vi "ClassPanel.vi"(8 "error in (no error)":errorcluster caption="entrée d'erreur (pas d'erreur)", 11 "MultiHarp150.lvclass":refnum<class "MultiHarp150.lvclass">) -> (0 "error out":errorcluster caption="sortie d'erreur", 3 "MultiHarp150.lvclass Out":refnum<class "MultiHarp150.lvclass">)   [LabVIEW 2019, in "MultiHarp150.lvclass"]
uses:
  MultiHarp150.lvclass
  C:/Programmes Labview/LabscanV1A/DevicesClass/BaseDevice/BaseDevice.lvclass
  <userlib>/MultiHarp150/MH_InputChannel_LS.ctl
  <userlib>/MultiHarp150/MH_MeasMode.ctl
  <userlib>/MultiHarp150/MH_RefSource.ctl
  <userlib>/MultiHarp150/UIThread/MH_SetInpChanData.ctl
  <userlib>/MultiHarp150/UIThread/MH_SetInpChanCmds.ctl
  MultiHarp150.lvclass/MultiHarp150.ctl
  BaseDevice/ClassQueueMess.ctl
  MultiHarp150_Func.ctl
  BaseDevice/Accessor/GetClassEvent.vi
  <vilib>/Utility/error.llb/Error Cluster From Error Code.vi
  <vilib>/ErrorRing/Error Ring.xnode
panel:
  out "ClearRef":refnum<vi>
  in  "Con/Disc.":bool
  out "Rate Avg Data":i32[][](array[numeric])
  out "Avg ref":refnum<vi>
  out "RtGrphAct":bool
  out "ViRef":refnum<vi>
  out "Graph":refnum<vi>
  out "Dat":refnum<vi>
  out "Rate Data":i32[][](array[numeric])
  out "binsteps":i32
  out "SetInpChan":T1[](array[typedef])
  out "DevIdx":i32
  in  "MH Tabs":enum32{"Main", "Settings", "Channels"}(tab)
  in  "Halt":bool
  out "Timeleft (ms)":dbl=60.0 caption="TimeLeft(ms)"
  in  "Rd.Cnt\nAcqu.":bool
  in  "ClearGrp":bool
  in  "AcqOffset (ns)":i32 caption="Offset (ns)" min=-1000000 max=100000000 step=1
  in  "Acqu. Time (ms)":i32=60 min=1 step=1
  out "SyncRate (CPS)":i32=60 format="%^.0e"
  in  "Clear Graph":bool caption="Clear\nGraph"
  in  "Save Data":bool caption="Save\nHist."
  in  "AquireHist":bool caption="MiseAJour"
  in  "Contin.\nAcqu.":bool
  out "OverFlow":bool caption="Ovrflw:"
  out "Count Rates":i32[](array[numeric]) format="%#.0f"
  in  "Rate Graph":bool
  in  "Read Cont.":bool
  out "AllHistoStats":T3(array[cluster]) {"MaxTime 2" format="%.3e"; "MaxTime" format="%.3e"; "HistRate (CPS)" format="%#.3f"; "TotalCount" format="%#.1f"}
  in  "Stats Ch":u16(ring) caption="Ch" items=["1", "2", "3", "4", "Sum", ""]
  in  "Binning":T4(ring) caption="Resol. (ps)"
  in  "OvlLevel":u32=4294967295 caption="Overload.Lvl" min=1 step=1
  in  "Stop Ovl.":bool
  in  "HistoLength":T5(ring)=enum."65536" caption="Num Bins"
  in  "SyncDivider":i32(ring) caption="Divider" items=["1", "2", "4", "8", "16"]
  in  "SyncEdge":i32(ring) caption="Edge" items=["falling", "rising"]
  in  "SyncLevel":i32=-100 caption="Level (mV)" min=-1200 max=1200 step=1
  in  "SyncOffset":i32 caption="Offset (ps)" min=-100000 max=100000 step=5
  in  "UseDeadTime":bool caption="Use DT."
  in  "SyncDeadTime":i32=1000 caption="Dead T. (ps)" min=800 max=160000 step=1
  in  "Panel Refresh":u32=400 caption="Panel Refresh (ms)" min=200 max=10000 step=200
  in  "Ref Source":T6
  in  "Mode":T7 items=["HIST"=0, "T2"=2, "T3"=3]
  in  "Graph #":i32 min=0 max=256 step=1
  in  "Channels":T8[](array[typedef]) {"DeadTime" min=800 max=160000 step=1; "Edge" items=["falling", "rising"]; "Offset" min=-100000 max=100000 step=5; "Level" min=-1200 max=1200 step=1}
  in  "MainProgQ":refnum<queue>
  in  "MainProgQEvent":refnum<user-event>
  in  "Acq":bool
  in  "Stop":bool
  out "Init Program":bool
  # "MultiHarp 150"
  # "this MUST labeled with class name"
  # "this MUST be present and labeled \"Stop\" and \"Acq\""
  # "Single Acq"
  # "Sync Channel"
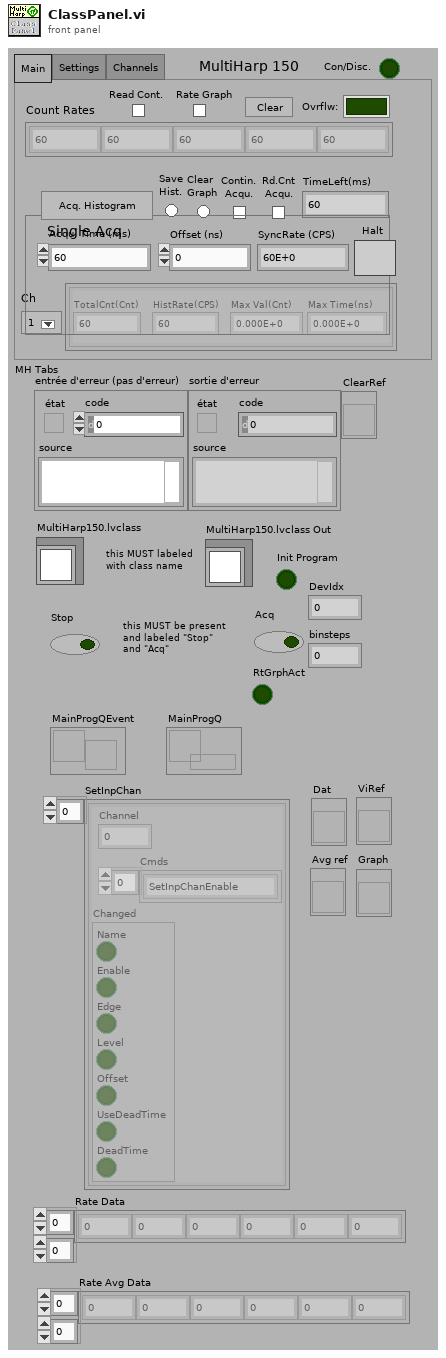
[diagram p1: front panel]
types:
  T1 = typedef "MH_SetInpChanData.ctl" = cluster{"Channel":i32, "Cmds":T2[], "Changed":cluster{"Name":bool, "Enable":bool, "Edge":bool, "Level":bool, "Offset":bool, "UseDeadTime":bool, "DeadTime":bool}}
  T2 = typedef "MH_SetInpChanCmds.ctl" = enum16{"SetInpChanEnable", "SetInpChanOffset", "SetInpChanDeadTime", "SetInpChanTrg"}
  T3 = cluster{"TotalCount":dbl, "HistRate (CPS)":dbl, "MaxTime 2":dbl, "MaxTime":dbl}[]
  T4 = enum16{"5", "10", "20", "40", "80", "160", "320", "640", "1280", "2560", "5120", "10240", "20480", "40960", "81920", "163840", "327680", "655360", "1310720", "2621440", "5242880", "10485760", "20971520", "41943040"}
  T5 = enum16{"1024", "2048", "4096", "8192", "16384", "32768", "65536"}
  T6 = typedef "MH_RefSource.ctl" = enum16{"INTERNAL", "EXTERNAL_10MHZ", "WR_MASTER_GENERIC", "WR_SLAVE_GENERIC", "WR_GRANDM_GENERIC", "EXTN_GPS_PPS", "EXTN_GPS_PPS_UART", "WR_MASTER_MHARP", "WR_SLAVE_MHARP", "WR_GRANDM_MHARP"}
  T7 = typedef "MH_MeasMode.ctl" = i32
  T8 = typedef "MH_InputChannel_LS.ctl" = cluster{"Name":string, "Enable":bool, "Edge":i32, "Level":i32, "Offset":i32, "UseDeadTime":bool, "DeadTime":i32}
  T9 = enum32{"Invalid", "Standard", "Closed", "Hidden", "Minimized", "Maximized"}
  T10 = typedef "MultiHarp150.lvclass/MultiHarp150_Func.ctl" = enum16{"ReadHistogram (Ph)", "ReadT2 (Ph)", "ReadT3 (Ph)", "ReadCount (Ph)"}
  T11 = enum16{"Enable", "Disable", "DisAndGrayed", "ReinitToDefVal", "EnumElementsArr"}
  T12 = cluster{dbl, "Panel Refresh":u32, "Rate Data Out":i32[][]}
  T13 = typedef "ClassQueueMess.ctl" = u16
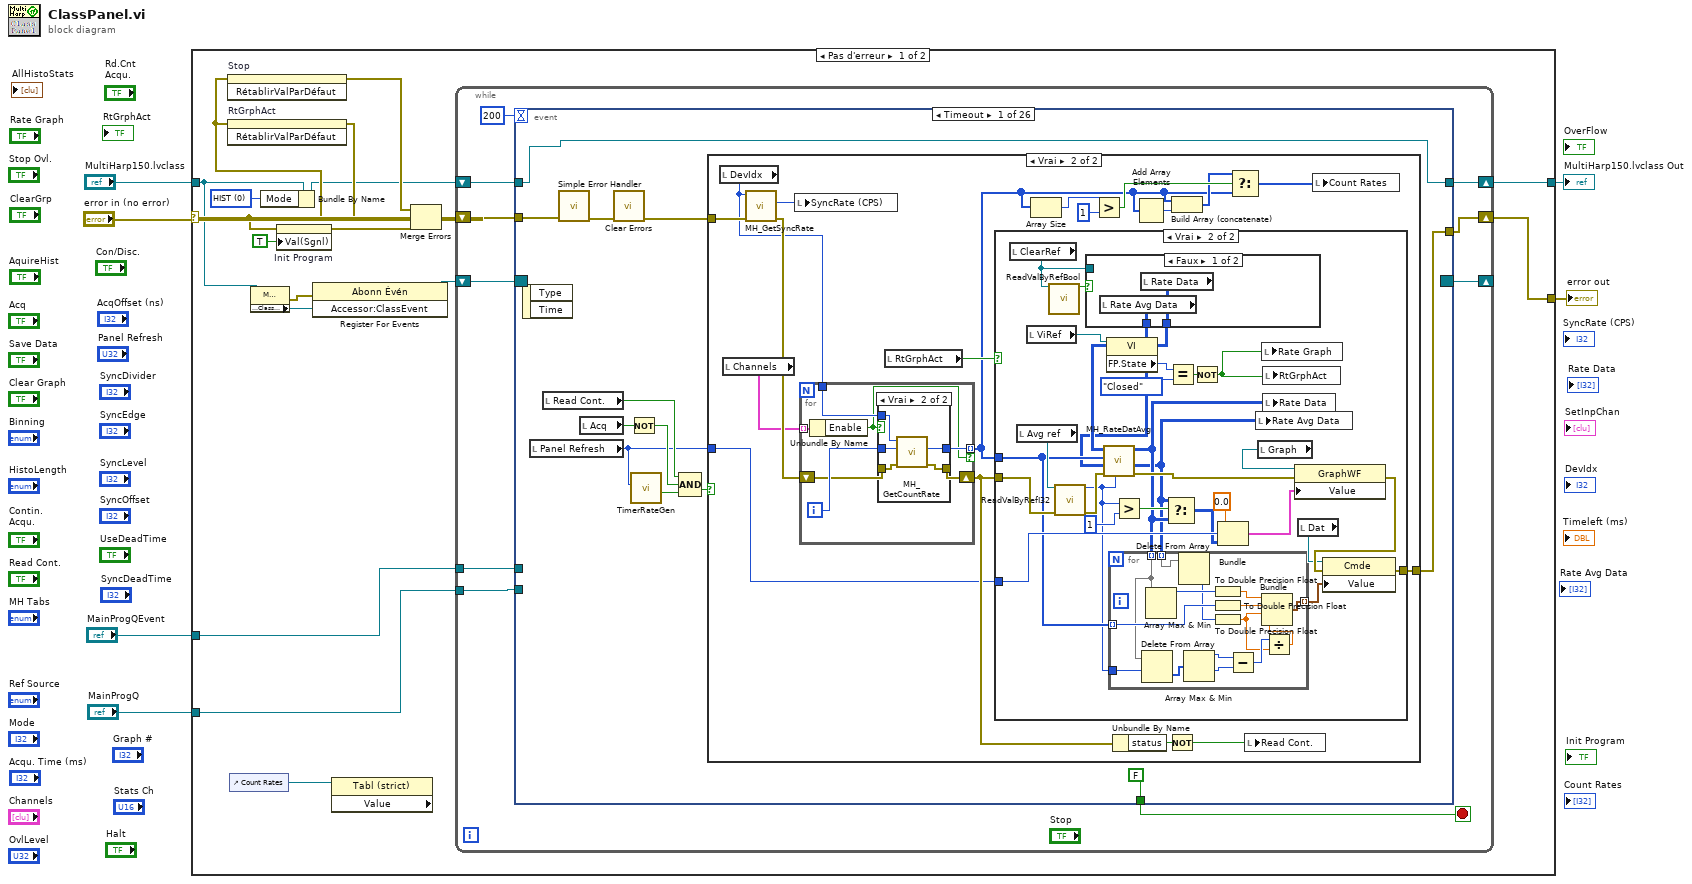
[diagram p0: block diagram]
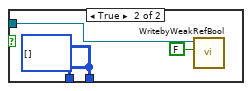
[diagram p4: hidden frame]
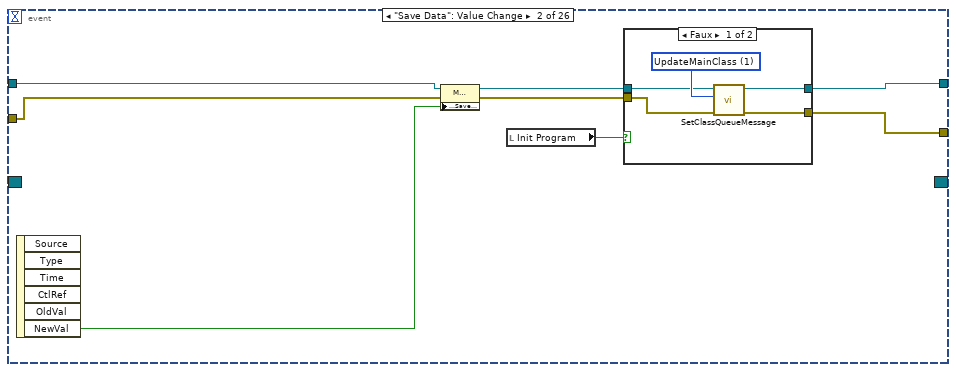
[diagram p6: hidden frame]
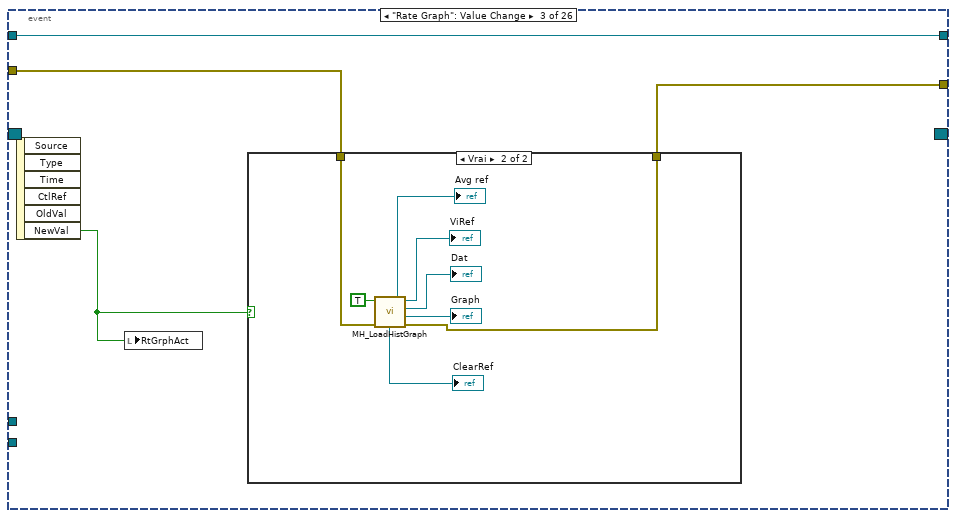
[diagram p8: hidden frame]
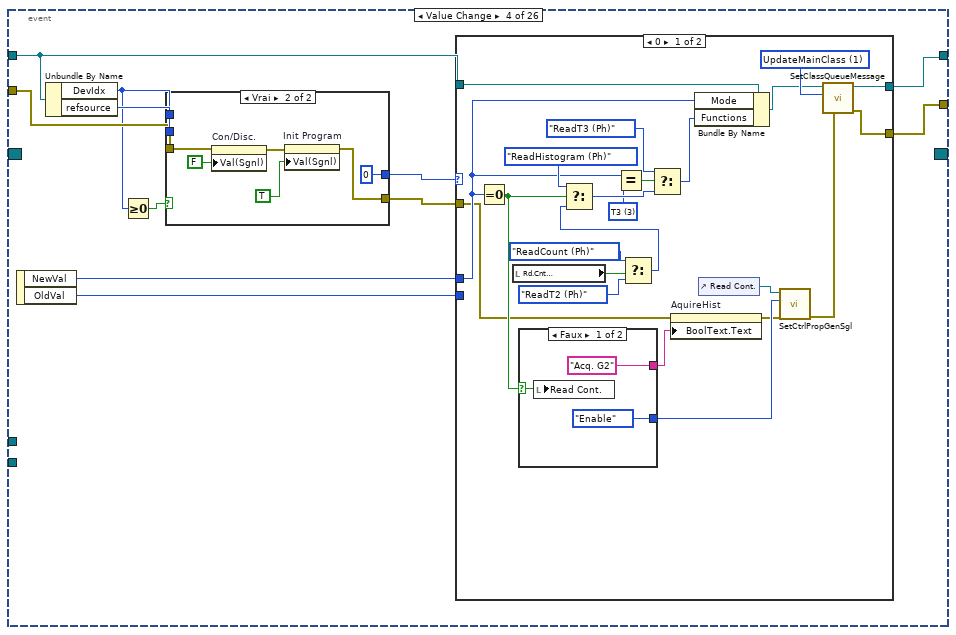
[diagram p10: hidden frame]
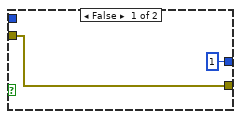
[diagram p11: hidden frame]
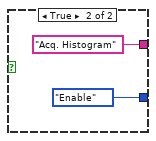
[diagram p12: hidden frame]
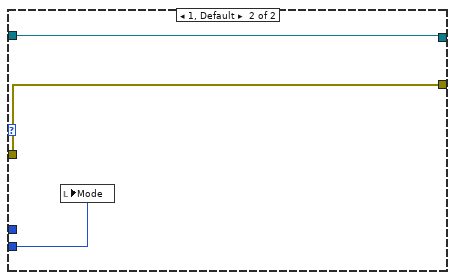
[diagram p13: hidden frame]
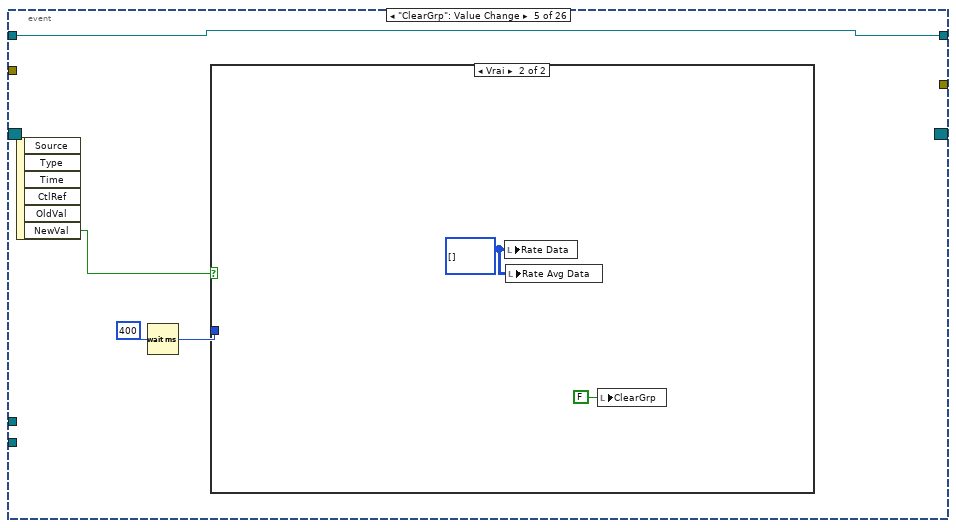
[diagram p14: hidden frame]
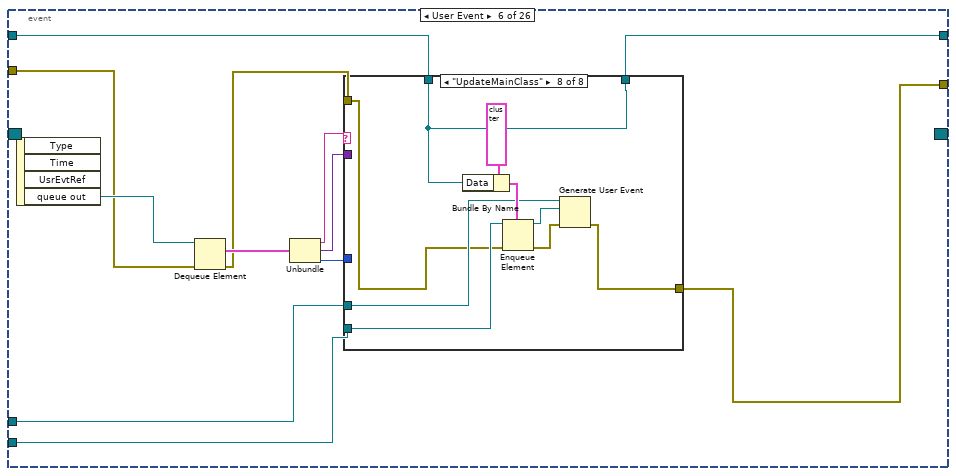
[diagram p16: hidden frame]
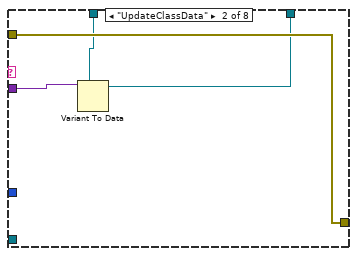
[diagram p18: hidden frame]
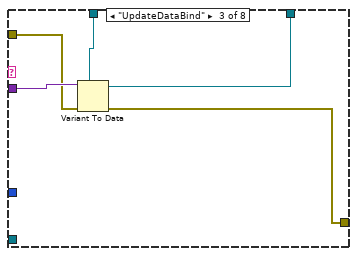
[diagram p19: hidden frame]
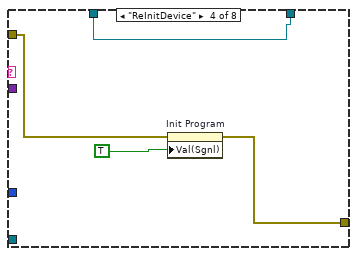
[diagram p20: hidden frame]
diagram:
  n1 = case shown="Pas d'erreur" "error in (no error)" {
    selector: "error in (no error)" -> [w11 w744]
    tunnel: [w23 w744] -> w5
    tunnel: "MultiHarp150.lvclass" -> [w19 w743]
    tunnel: [w22 w743] -> w3
    tunnel: "MainProgQEvent" -> [w17 _]
    tunnel: "MainProgQ" -> [w16 _]
    frame No Error {
      w8 = T7 0 items=["HIST"=0, "T2"=2, "T3"=3] ("Mode")
      n2 = invoke on="Stop" class="Bool (strict)" method="RétablirValParDéfaut"(error in=w11) -> (error out=w14:errorcluster)  [unwired: 2 in, 2 out]
      n3 = invoke on="RtGrphAct" class="Bool (strict)" method="RétablirValParDéfaut"(error in=w11) -> (error out=w13:errorcluster)  [unwired: 2 in, 2 out]
      n4 = control-ref of="Count Rates"() -> (w7:refnum<vi>)
      n5 = property class="MultiHarp150.lvclass"(reference=w19) -> (error out=w21:errorcluster, "Accessor:ClassEvent"=w20:refnum<user-event>)  [unwired: 1 in, 1 out]
      n6 = Bundle By Name(cluster=w19, "Mode"=w8) -> (w9:refnum<class "MultiHarp150.lvclass">)
      n7 = property on="Init Program" class="Bool (strict)"(error in=w11, "Val(Sgnl)"=TRUE ("Valeur (Signalisation)")) -> (error out=w10:errorcluster)  [unwired: 1 in, 1 out]
      n8 = register-events(error in=w21, w20) -> (reference out=w18:refnum<event-registration>)  [unwired: 1 in, 1 out]
      n9 = property class="Tabl (strict)" props=["Value"](reference=w7) -> ()  [unwired: 1 in, 3 out]
      n10 = Merge Errors(w14, w13, w10) -> (w15:errorcluster)
      n11 = while {
        shift-right: [w31] -> w23
        shift-left: w15 -> [w32]
        shift-right: [w29] -> w22
        shift-left: w9 -> [w30]
        shift-right: [w27] -> _
        shift-left: w18 -> [w28]
        tunnel: w17 -> [w26]
        tunnel: w16 -> [w25]
        stop <- w24 stop-if-true
        n12 = event shown="[0] Timeout" {
          selector: w28 -> [_ _ _ _ _ _ _ _ _ _ _ _ _ _ _ _ _ _ _ _ _ _ _ _ _ _]
          dyn-events: [_ _ _ _ _ _ _ _ _ _ _ _ _ _ _ _ _ _ _ _ _ _ _ _ _ _] -> w27
          timeout: 200 -> [_ _ _ _ _ _ _ _ _ _ _ _ _ _ _ _ _ _ _ _ _ _ _ _ _ _]
          tunnel: w32 -> [w44 w133 w144 w160 _ w212 w260 w316 w326 w346 w362 w380 w392 w410 _ w424 w488 w505 w535 w567 w591 w609 w625 w675 w702 w725]
          tunnel: [w41 w128 w143 w162 _ w216 w259 w315 w321 w341 w359 w373 w388 w413 _ w425 w489 w501 w531 w563 w586 w601 w624 w672 w704 w720] -> w31
          tunnel: w30 -> [w36 w134 w145 w155 w205 w222 w258 w317 w329 w347 w358 w381 w393 w408 w416 w427 w494 w496 w528 w560 w584 w600 w627 w674 w703 w726]
          tunnel: [FALSE _ _ _ _ _ _ _ _ _ _ _ _ _ _ _ _ _ _ _ _ _ _ TRUE FALSE _] -> w24
          tunnel: [w36 w129 w145 w164 w205 w215 w257 w314 w323 w343 w361 w375 w390 w414 w416 w421 w490 w502 w532 w565 w588 w606 w628 w673 w703 w719] -> w29
          tunnel: w26 -> [_ _ _ _ _ w214 _ _ _ _ _ _ _ _ _ _ _ _ _ _ _ _ w623 _ _ _]
          tunnel: w25 -> [_ _ _ _ _ w213 _ _ _ _ _ _ _ _ _ _ _ _ _ _ _ _ w622 _ _ _]
          event Timeout {
            n13 = event-data() -> ()  [unwired: 1 in, 2 out]
            n14 = local read "Panel Refresh"() -> (w35:u32)
            n15 = local read "Read Cont."() -> (w37:bool)
            n16 = call <vilib>:"Simple Error Handler.vi"("error in (no error)"=w44) -> ("error out"=w43:errorcluster)  [unwired: 4 in, 4 out]
            n17 = local read "Acq"() -> (w39:bool)
            n18 = call <vilib>:"Clear Errors.vi"("error in (no error)"=w43) -> ("error out"=w42:errorcluster)  [unwired: 5 in, 1 out]
            n19 = Not(x=w39) -> (.not. x?=w38:bool)
            n20 = call <userlib>:"TimerRateGen.vi"("Refresh(ms)"=w35) -> ("updated?"=w34:bool)  [unwired: 8 in, 2 out]
            n21 = Compound Arithmetic op=AND ("Opérateur arithmétique")(w37, w38, w34) -> (w40:bool)
            n22 = case shown="Vrai" w40 {
              tunnel: w42 -> [w46 w64]
              tunnel: [w46 w60] -> w41
              tunnel: w35 -> [_ w58]
              frame False {
              }
              frame True {
                n23 = local read "DevIdx"() -> (w48:i32)
                n24 = local read "Channels"() -> (w47:T8[])
                n25 = call <userlib>:"MH_GetSyncRate.vi"("error in (no error)"=w64, "devidx"=w48) -> ("error out"=w56:errorcluster, "syncrate"=w59:i32)  [unwired: 7 in, 1 out]
                n26 = local write "SyncRate (CPS)"(w59) -> ()
                n27 = for {
                  tunnel: w47 -> [w120] mode=indexing
                  tunnel: w48 -> [w118]
                  shift-right: [w116] -> w61
                  shift-left: w56 -> [w117]
                  tunnel: [w115] -> w50 mode=indexing if=w114
                  i -> [w119]
                  n28 = Unbundle By Name(w120) -> ("Enable"=w114:bool)
                  n29 = case shown="Vrai" w114 {
                    tunnel: w119 -> [_ w126]
                    tunnel: w118 -> [_ w122]
                    tunnel: w117 -> [w121 w125]
                    tunnel: [w121 w124] -> w116
                    tunnel: [_ w123] -> w115
                    frame False {
                    }
                    frame True {
                      n30 = call <userlib>:"MH_GetCountRate.vi"("error in (no error)"=w125, "Channel"=w126, "devidx"=w122) -> ("error out"=w124:errorcluster, "rate"=w123:i32)  [unwired: 6 in, 1 out]
                    }
                  }
                }
                n31 = local read "RtGrphAct"() -> (w57:bool)
                n32 = case shown="Vrai" w57 {
                  tunnel: w61 -> [w65 w79]
                  tunnel: [w65 w90] -> w60
                  tunnel: w50 -> [_ w77]
                  tunnel: w58 -> [_ w81]
                  frame False {
                  }
                  frame True {
                    n33 = local read "ClearRef"() -> (w71:refnum<vi>)
                    n34 = local read "Avg ref"() -> (w80:refnum<vi>)
                    n35 = local read "ViRef"() -> (w86:refnum<vi>)
                    n36 = call <userlib>:"ReadValByRefBool.vi"("Control Ref"=w71) -> ("Valeur"=w72:bool)  [unwired: 13 in, 1 out]
                    n37 = call <userlib>:"ReadValByRefI32.vi"("Control Ref"=w80, "error in"=w79) -> ("Valeur"=w66:i32, "error out"=w78:errorcluster)  [unwired: 12 in]
                    n38 = case shown="Faux" w72 {
                      tunnel: w71 -> [_ w96]
                      tunnel: [w95 w97] -> w69
                      tunnel: [w94 w97] -> w68
                      frame False {
                        n39 = local read "Rate Avg Data"() -> (w94:i32[][])
                        n40 = local read "Rate Data"() -> (w95:i32[][])
                      }
                      frame True {
                        w97 = i32[][] [] ("Rate Data")
                        n41 = call <userlib>:"WritebyWeakRefBool.vi"("Valeur"=FALSE, "Control Ref"=w96) -> ()  [unwired: 9 in, 1 out]
                      }
                    }
                    n42 = call <userlib>:"MH_RateDatAvg.vi"("Avg Val"=w66, "error in (no error)"=w78, "RateAvg Data"=w68, "Count Rates"=w77, "Rate Data"=w69) -> ("error out"=w76:errorcluster, "RateAvg Data Out"=w67:i32[][], "Rate Data Out"=w70:i32[][])  [unwired: 4 in]
                    n43 = property class="VI"(reference=w86) -> ("FP.State"=w85:T9)  [unwired: 1 in, 2 out]
                    n44 = for {
                      tunnel: w70 -> [w106] mode=indexing
                      tunnel: w77 -> [w110] mode=indexing
                      tunnel: [w113] -> w89 mode=indexing
                      tunnel: w67 -> [w108] mode=indexing
                      tunnel: w66 -> [w105]
                      n45 = Delete From Array(array=w106, length=w105) -> (deleted portion=w104:i32[])  [unwired: 1 in, 1 out]
                      n46 = Array Max & Min(array=w106) -> (max value=w109:i32)  [unwired: 3 out]
                      n47 = Delete From Array(array=w108) -> (deleted portion=w107:i32)  [unwired: 2 in, 1 out]
                      n48 = Array Max & Min(array=w104) -> (max value=w103:i32, min value=w102:i32)  [unwired: 2 out]
                      n49 = To Double Precision Float(number=w109) -> (double precision float=w112:dbl)
                      n50 = To Double Precision Float(number=w110) -> (double precision float=w111:dbl)
                      n51 = To Double Precision Float(number=w107) -> (double precision float=w100:dbl)
                      n52 = Subtract(x=w103, y=w102) -> (x-y=w101:i32)
                      n53 = Divide(x=w101, y=w100) -> (x/y=w99:dbl)
                      n54 = Bundle(w112, w111, w100, w99) -> (w113:cluster{dbl, dbl, dbl, dbl})  [unwired: 1 in]
                    }
                    n55 = Greater?(x=w66, y=1) -> (0:w74:bool)
                    n56 = Select(t=w67, s=w74, f=w70) -> (s? t:f=w73:i32[][])
                    n57 = Equal?(x=w85, y=T9."Closed") -> (x = y?=w83:bool)
                    n58 = Not(x=w83) -> (.not. x?=w82:bool)
                    n59 = Bundle(0.0, "Panel Refresh"=w81, "Rate Data Out"=w73) -> (w92:T12)  [unwired: 1 in]
                    n60 = local write "Rate Avg Data"(w67) -> ()
                    n61 = local read "Graph"() -> (w88:refnum<vi>)
                    n62 = local write "Rate Graph"(w82) -> ()
                    n63 = local write "RtGrphAct"(w82) -> ()
                    n64 = local write "Rate Data"(w70) -> ()
                    n65 = property class="GraphWF"(reference=w88, error in=w76, "Value"=w92) -> (error out=w91:errorcluster)  [unwired: 1 out]
                    n66 = local read "Dat"() -> (w87:refnum<vi>)
                    n67 = property class="Cmde"(reference=w87, error in=w91, "Value"=w89) -> (error out=w90:errorcluster)  [unwired: 1 out]
                  }
                }
                n68 = Array Size(array=w50) -> (size(s)=w55:i32)
                n69 = Greater?(x=w55, y=1) -> (0:w52:bool)
                n70 = Unbundle By Name(w61) -> ("status"=w63:bool)
                n71 = Add Array Elements(numeric array=w50) -> (sum=w53:i32)
                n72 = Not(x=w63) -> (.not. x?=w62:bool)
                n73 = Build Array (concatenate)(w50, w53) -> (w51:i32[])
                n74 = Select(t=w51, s=w52, f=w50) -> (s? t:f=w49:i32[])
                n75 = local write "Read Cont."(w62) -> ()
                n76 = local write "Count Rates"(w49) -> ()
              }
            }
          }
          event "Save Data": Value Change {
            n77 = event-data() -> ("NewVal"=w132:bool)  [unwired: 1 in, 5 out]
            n78 = property class="MultiHarp150.lvclass"(reference=w134, error in=w133, "Accessor:SaveArrDat"=w132) -> (reference out=w131:refnum<class "MultiHarp150.lvclass">, error out=w130:errorcluster)
            n79 = local read "Init Program"() -> (w127:bool)
            n80 = case shown="Faux" w127 {
              tunnel: w131 -> [w138 w141]
              tunnel: w130 -> [w137 w140]
              tunnel: [w136 w141] -> w129
              tunnel: [w135 w140] -> w128
              frame False {
                w139 = T13 1 items=["UpdateClassData", "UpdateMainClass"] ("Menu déroulant")
                n81 = call-dynamic "SetClassQueueMessage.vi"("ErrorIn(No Error)"=w137, "Menu déroulant"=w139, "DefaultDev.lvclass"=w138) -> ("sortie d'erreur"=w135:errorcluster, "DefaultDev.lvclass Out"=w136:refnum<class "MultiHarp150.lvclass">)  [unwired: 7 in]
              }
              frame True {
              }
            }
          }
          event "Rate Graph": Value Change {
            n82 = event-data() -> ("NewVal"=w142:bool)  [unwired: 1 in, 5 out]
            n83 = local write "RtGrphAct"(w142) -> ()
            n84 = case shown="Vrai" w142 {
              tunnel: w144 -> [w146 w152]
              tunnel: [w146 w151] -> w143
              frame False {
              }
              frame True {
                n85 = call <userlib>:"MH_LoadHistGraph.vi"("ErrIn(No Err)"=w152, "Rate Mode"=TRUE) -> ("ErrOut"=w151:errorcluster, "Graph"=→"Graph":refnum<vi>, "Dat"=→"Dat":refnum<vi>, "ViRef"=→"ViRef":refnum<vi>, "Avg ref"=→"Avg ref":refnum<vi>, "ClearRef"=→"ClearRef":refnum<vi>)  [unwired: 3 in, 1 out]
              }
            }
          }
          event Value Change {
            n86 = event-data() -> ("NewVal"=w158:T7, "OldVal"=w159:T7)  [unwired: 1 in]
            n87 = Unbundle By Name(w155) -> ("DevIdx"=w157:i32, "refsource"=w165:T6)
            n88 = Greater Or Equal To 0?(x=w157) -> (x >= 0?=w156:bool)
            n89 = case shown="Vrai" w156 {
              tunnel: w165 -> [_ _]
              tunnel: [w166 w169] -> w163
              tunnel: [1 ("return type") 0 ("return type")] -> w161
              tunnel: w157 -> [_ _]
              tunnel: w160 -> [w166 w173]
              frame False {
              }
              frame True {
                n90 = property on="Con/Disc." class="Bool (strict)"(error in=w173, "Val(Sgnl)"=FALSE ("Valeur (Signalisation)")) -> (error out=w171:errorcluster)  [unwired: 1 in, 1 out]
                n91 = property on="Init Program" class="Bool (strict)"(error in=w171, "Val(Sgnl)"=TRUE ("Valeur (Signalisation)")) -> (error out=w169:errorcluster)  [unwired: 1 in, 1 out]
              }
            }
            n92 = case shown="0" w161 {
              tunnel: w155 -> [w196 w204]
              tunnel: [w193 w204] -> w164
              tunnel: w163 -> [w179 w203]
              tunnel: [w192 w203] -> w162
              tunnel: w158 -> [w188 _]
              tunnel: w159 -> [_ w202]
              frame 0 {
                w187 = T7 3 items=["HIST"=0, "T2"=2, "T3"=3] ("y")
                w195 = T13 1 items=["UpdateClassData", "UpdateMainClass"] ("Menu déroulant")
                n93 = Equal To 0?(x=w188) -> (x = 0?=w183:bool)
                n94 = local read "Rd.Cnt\nAcqu."() -> (w177:bool)
                n95 = case shown="Faux" w183 {
                  selector: w183 -> [w199 _]
                  tunnel: [T11."Enable" ("Énum") T11."Enable" ("Énum")] -> w182
                  tunnel: ["Acq. G2" ("Texte booléen.Texte") "Acq. Histogram" ("Texte booléen.Texte")] -> w178
                  frame False {
                    n96 = local write "Read Cont."(w199) -> ()
                  }
                  frame True {
                  }
                }
                n97 = Equal?(x=w188, y=w187) -> (x = y?=w189:bool)
                n98 = Select(t=MultiHarp150_Func."ReadCount (Ph)" ("Functions"), s=w177, f=MultiHarp150_Func."ReadT2 (Ph)" ("Functions")) -> (s? t:f=w174:T10)
                n99 = Select(t=MultiHarp150_Func."ReadHistogram (Ph)" ("Functions"), s=w183, f=w174) -> (s? t:f=w190:T10)
                n100 = Select(t=MultiHarp150_Func."ReadT3 (Ph)" ("Functions"), s=w189, f=w190) -> (s? t:f=w185:T10)
                n101 = property on="AquireHist" class="Bool (strict)"(error in=w179, "BoolText.Text"=w178) -> (error out=w180:errorcluster)  [unwired: 1 in, 1 out]
                n102 = Bundle By Name(cluster=w196, "Mode"=w188, "Functions"=w185) -> (w194:refnum<class "MultiHarp150.lvclass">)
                n103 = control-ref of="Read Cont."() -> (w184:refnum<vi>)
                n104 = call <userlib>:"SetCtrlPropGenSgl.vi"("Error in"=w180, "Énum"=w182, "Controls"=w184) -> ("Error out"=w181:errorcluster)  [unwired: 3 in, 1 out]
                n105 = call-dynamic "SetClassQueueMessage.vi"("ErrorIn(No Error)"=w181, "Menu déroulant"=w195, "DefaultDev.lvclass"=w194) -> ("sortie d'erreur"=w192:errorcluster, "DefaultDev.lvclass Out"=w193:refnum<class "MultiHarp150.lvclass">)  [unwired: 7 in]
              }
              frame 1, Default {
                n106 = local write "Mode"(w202) -> ()
              }
            }
          }
          event "ClearGrp": Value Change {
            n107 = event-data() -> ("NewVal"=w208:bool)  [unwired: 1 in, 5 out]
            n108 = Wait (ms)(milliseconds to wait=u32 400 ("attente (ms)")) -> (millisecond timer value=w207:u32)
            n109 = case shown="Vrai" w208 {
              tunnel: w207 -> [_ _]
              frame False {
              }
              frame True {
                w209 = i32[][] [] ("Rate Data")
                n110 = local write "Rate Data"(w209) -> ()
                n111 = local write "Rate Avg Data"(w209) -> ()
                n112 = local write "ClearGrp"(FALSE ("ClearGrp")) -> ()
              }
            }
          }
          event User Event {
            n113 = event-data() -> ("queue out"=w220:refnum<queue>)  [unwired: 1 in, 3 out]
            n114 = Dequeue Element(queue=w220, error in (no error)=w212) -> (element=w221:cluster{"Message":string, "Data":variant, i32}, error out=w211:errorcluster)  [unwired: 1 in, 2 out]
            n115 = Unbundle(w221) -> ("Message"=w219:string, "Data"=w218:variant, w217:i32)
            n116 = case shown="\"UpdateMainClass\"" w219 {
              tunnel: w211 -> [w224 w228 w230 w235 w239 w242 w246 w249]
              tunnel: w218 -> [_ w227 w233 _ _ _ _ _]
              tunnel: w222 -> [w223 w226 w232 w237 w241 w243 w247 w252]
              tunnel: [w223 w225 w231 w237 w241 w243 w247 w252] -> w215
              tunnel: [w224 w228 w229 w234 w238 w242 w246 w248] -> w216
              tunnel: w217 -> [_ _ _ _ _ _ _ _]
              tunnel: w214 -> [_ _ _ _ _ _ _ w251]
              tunnel: w213 -> [_ _ _ _ _ _ _ w250]
              frame Default {
              }
              frame "UpdateClassData" {
                n117 = Variant To Data(type=w226, Variant=w227) -> (data=w225:refnum<class "MultiHarp150.lvclass">)  [unwired: 1 in, 1 out]
              }
              frame "UpdateDataBind" {
                n118 = Variant To Data(error in=w230, type=w232, Variant=w233) -> (data=w231:refnum<class "MultiHarp150.lvclass">, error out=w229:errorcluster)
              }
              frame "ReInitDevice" {
                n119 = property on="Init Program" class="Bool (strict)"(error in=w235, "Val(Sgnl)"=TRUE ("Valeur (Signalisation)")) -> (error out=w234:errorcluster)  [unwired: 1 in, 1 out]
              }
              frame "Disconnect Device" {
                n120 = property on="Con/Disc." class="Bool (strict)"(error in=w239, "Val(Sgnl)"=FALSE ("Valeur (Signalisation)")) -> (error out=w238:errorcluster)  [unwired: 1 in, 1 out]
              }
              frame "MeasDone" {
              }
              frame "ShowDiag" {
                n121 = control-ref of="This VI"() -> (w245:refnum<vi>)
                n122 = call <userlib>:"AnimExecGen.vi"("Animer l'exécution ?"=TRUE, "ViRef"=w245) -> ()  [unwired: 9 in, 1 out]
              }
              frame "UpdateMainClass" {
                n123 = Bundle By Name(cluster=cluster{"Message":string, "Data":variant, i32} {"Message"="", "Data"=variant, 0} ("élément"), "Data"=w252) -> (w253:cluster{"Message":string, "Data":variant, i32})
                n124 = Enqueue Element(queue=w250, element=w253, error in (no error)=w249) -> (queue out=w256:refnum<queue>, error out=w255:errorcluster)  [unwired: 1 in, 1 out]
                n125 = Generate User Event(user event=w251, event data cluster=w256, error in=w255) -> (error out=w248:errorcluster)  [unwired: 1 in, 1 out]
              }
            }
          }
          event "Init Program": Value Change {
            n126 = event-data() -> ("NewVal"=w261:bool)  [unwired: 1 in]
            n127 = case shown="Vrai" w261 {
              tunnel: w260 -> [w263 w302]
              tunnel: [w263 w289] -> w259
              tunnel: w258 -> [w262 w272]
              tunnel: [w262 w270] -> w257
              frame False {
              }
              frame True {
                n128 = xnode "Menu déroulant d'erreurs"() -> ("sortie d'erreur"=w266:errorcluster)
                n129 = Unbundle By Name(w272) -> ("Mode"=w286:T7, "refsource"=w284:T6, "Panel Refresh"=w285:dbl, "SyncDivider"=w281:i32, "SyncOffset"=w288:i32, "SyncEdge"=w296:i32, "SyncDeadTime"=w280:i32, "Binning"=w279:T4, "HistoLength"=w278:T5, "HistoOffset(ns)"=w275:i32, "OvlLevel"=w277:u32, "Channels"=w301:T8[], "SyncLevel"=w282:i32, "Stop Ovl."=w283:bool, "UseDeadTime"=w287:bool, "AcquTime(ms)"=w276:i32)
                n130 = for {
                  N: 8 -> [_]
                  tunnel: [w310] -> w265
                  tunnel: [w309] -> _
                  tunnel: [w311] -> w299
                  tunnel: w302 -> [w308]
                  i -> [w311]
                  stop <- w310 continue-if-true
                  n131 = call <userlib>:"MH_OpenDevice.vi"("error in (no error)"=w308, "devidx"=w311) -> ("error out"=w310:errorcluster, "serial"=w309:string)  [unwired: 7 in, 1 out]
                }
                n132 = local write "Mode"(w286) -> ()
                n133 = local write "Ref Source"(w284) -> ()
                n134 = local write "Panel Refresh"(w285) -> ()
                n135 = Select(t=w266, s=w265, f=w265) -> (s? t:f=w264:errorcluster)
                n136 = local write "SyncLevel"(w282) -> ()
                n137 = local write "Stop Ovl."(w283) -> ()
                n138 = local write "UseDeadTime"(w287) -> ()
                n139 = local write "Acqu. Time (ms)"(w276) -> ()
                n140 = local write "Channels"(w301) -> ()
                n141 = Select(t=-1, s=w264, f=w299) -> (s? t:f=w271:i32)
                n142 = call <userlib>:"MH_Initialize.vi"("error in (no error)"=w264, "refsource"=w284, "mode"=w286, "devidx"=w271) -> ("error out"=w269:errorcluster)  [unwired: 6 in, 1 out]
                n143 = property on="Save Data" class="Bool (strict)"(error in=w269, "Val(Sgnl)"=TRUE ("Valeur (Signalisation)")) -> (error out=w268:errorcluster)  [unwired: 1 in, 1 out]
                n144 = Bundle By Name(cluster=w272, "DevIdx"=w271) -> (w270:refnum<class "MultiHarp150.lvclass">)
                n145 = property on="SyncDivider" class="MDér (strict)"(error in=w268, "Val(Sgnl)"=w281) -> (error out=w295:errorcluster)  [unwired: 1 in, 1 out]
                n146 = property on="SyncOffset" class="NumNb (strict)"(error in=w295, "Val(Sgnl)"=w288) -> (error out=w294:errorcluster)  [unwired: 1 in, 1 out]
                n147 = property on="SyncEdge" class="MDér (strict)"(error in=w294, "Val(Sgnl)"=w296) -> (error out=w293:errorcluster)  [unwired: 1 in, 1 out]
                n148 = property on="SyncDeadTime" class="NumNb (strict)"(error in=w293, "Val(Sgnl)"=w280) -> (error out=w292:errorcluster)  [unwired: 1 in, 1 out]
                n149 = property on="SetInpChan" class="Tabl (strict)"(error in=w292, "Val(Sgnl)"=T1[] [{"Channel"=0, "Cmds"=[enum."SetInpChanEnable", enum."SetInpChanTrg", enum."SetInpChanOffset", enum."SetInpChanDeadTime"], "Changed"={"Name"=FALSE, "Enable"=FALSE, "Edge"=FALSE, "Level"=FALSE, "Offset"=FALSE, "UseDeadTime"=FALSE, "DeadTime"=FALSE}}, {"Channel"=1, "Cmds"=[enum."SetInpChanEnable", enum."SetInpChanTrg", enum."SetInpChanOffset", enum."SetInpChanDeadTime"], "Changed"={"Name"=FALSE, "Enable"=FALSE, "Edge"=FALSE, "Level"=FALSE, "Offset"=FALSE, "UseDeadTime"=FALSE, "DeadTime"=FALSE}}, {"Channel"=2, "Cmds"=[enum."SetInpChanEnable", enum."SetInpChanTrg", enum."SetInpChanOffset", enum."SetInpChanDeadTime"], "Changed"={"Name"=FALSE, "Enable"=FALSE, "Edge"=FALSE, "Level"=FALSE, "Offset"=FALSE, "UseDeadTime"=FALSE, "DeadTime"=FALSE}}, {"Channel"=3, "Cmds"=[enum."SetInpChanEnable", enum."SetInpChanTrg", enum."SetInpChanOffset", enum."SetInpChanDeadTime"], "Changed"={"Name"=FALSE, "Enable"=FALSE, "Edge"=FALSE, "Level"=FALSE, "Offset"=FALSE, "UseDeadTime"=FALSE, "DeadTime"=FALSE}}] ("Valeur (Signalisation)")) -> (error out=w291:errorcluster)  [unwired: 1 in, 1 out]
                n150 = property on="Binning" class="Énum (strict)"(error in=w291, "Val(Sgnl)"=w279) -> (error out=w290:errorcluster)  [unwired: 1 in, 1 out]
                n151 = property on="HistoLength" class="Énum (strict)"(error in=w290, "Val(Sgnl)"=w278) -> (error out=w274:errorcluster)  [unwired: 1 in, 1 out]
                n152 = property on="AcqOffset (ns)" class="NumNb (strict)"(error in=w274, "Val(Sgnl)"=w275) -> (error out=w273:errorcluster)  [unwired: 1 in, 1 out]
                n153 = property on="OvlLevel" class="NumNb (strict)"(error in=w273, "Val(Sgnl)"=w277) -> (error out=w289:errorcluster)  [unwired: 1 in, 1 out]
              }
            }
          }
          event "Panel Refresh": Value Change {
            w313 = T13 1 items=["UpdateClassData", "UpdateMainClass"] ("Menu déroulant")
            n154 = event-data() -> ("NewVal"=w318:u32)  [unwired: 1 in, 5 out]
            n155 = Bundle By Name(cluster=w317, "Panel Refresh"=w318) -> (w312:refnum<class "MultiHarp150.lvclass">)
            n156 = call-dynamic "SetClassQueueMessage.vi"("ErrorIn(No Error)"=w316, "Menu déroulant"=w313, "DefaultDev.lvclass"=w312) -> ("sortie d'erreur"=w315:errorcluster, "DefaultDev.lvclass Out"=w314:refnum<class "MultiHarp150.lvclass">)  [unwired: 7 in]
          }
          event "SyncDivider": Value Change {
            n157 = event-data() -> ("NewVal"=w320:i32)  [unwired: 1 in, 5 out]
            n158 = local read "DevIdx"() -> (w327:i32)
            n159 = Power Of 2(x=w320) -> (2^x=w330:dbl)
            n160 = To Long Integer(number=w330) -> (32bit integer=w328:i32)
            n161 = Bundle By Name(cluster=w329, "SyncDivider"=w320) -> (w324:refnum<class "MultiHarp150.lvclass">)
            n162 = call <userlib>:"MH_SetSyncDiv.vi"("error in (no error)"=w326, "SyncDivider"=w328, "devidx"=w327) -> ("error out"=w325:errorcluster)  [unwired: 7 in, 1 out]
            n163 = flat-sequence {
              tunnel: w325 -> [w338]
              tunnel: [w338] -> w322
              frame #0 {
                n164 = Wait (ms)(milliseconds to wait=u32 100) -> ()  [unwired: 1 out]
              }
            }
            n165 = local read "Init Program"() -> (w319:bool)
            n166 = case shown="Faux" w319 {
              tunnel: w324 -> [w334 w336]
              tunnel: [w333 w336] -> w323
              tunnel: w322 -> [w332 w337]
              tunnel: [w331 w337] -> w321
              frame False {
                w335 = T13 1 items=["UpdateClassData", "UpdateMainClass"] ("Menu déroulant")
                n167 = call-dynamic "SetClassQueueMessage.vi"("ErrorIn(No Error)"=w332, "Menu déroulant"=w335, "DefaultDev.lvclass"=w334) -> ("sortie d'erreur"=w331:errorcluster, "DefaultDev.lvclass Out"=w333:refnum<class "MultiHarp150.lvclass">)  [unwired: 7 in]
              }
              frame True {
              }
            }
          }
          event "SyncOffset": Value Change {
            n168 = event-data() -> ("NewVal"=w345:i32)  [unwired: 1 in]
            n169 = local read "DevIdx"() -> (w348:i32)
            n170 = call <userlib>:"MH_SetSyncChannelOffset.vi"("error in (no error)"=w346, "Offset"=w345, "devidx"=w348) -> ("error out"=w342:errorcluster)  [unwired: 7 in, 1 out]
            n171 = Bundle By Name(cluster=w347, "SyncOffset"=w345) -> (w344:refnum<class "MultiHarp150.lvclass">)
            n172 = local read "Init Program"() -> (w340:bool)
            n173 = case shown="Faux" w340 {
              tunnel: w344 -> [w352 w354]
              tunnel: [w351 w354] -> w343
              tunnel: w342 -> [w350 w355]
              tunnel: [w349 w355] -> w341
              frame False {
                w353 = T13 1 items=["UpdateClassData", "UpdateMainClass"] ("Menu déroulant")
                n174 = call-dynamic "SetClassQueueMessage.vi"("ErrorIn(No Error)"=w350, "Menu déroulant"=w353, "DefaultDev.lvclass"=w352) -> ("sortie d'erreur"=w349:errorcluster, "DefaultDev.lvclass Out"=w351:refnum<class "MultiHarp150.lvclass">)  [unwired: 7 in]
              }
              frame True {
              }
            }
          }
          event "SyncEdge": Value Change {
            n175 = event-data() -> ("NewVal"=w363:i32)  [unwired: 1 in]
            n176 = local read "SyncLevel"() -> (w364:i32)
            n177 = local read "DevIdx"() -> (w365:i32)
            n178 = call <userlib>:"MH_SetSyncEdgeTrg.vi"("error in (no error)"=w362, "edge"=w363, "level"=w364, "devidx"=w365) -> ("error out"=w360:errorcluster)  [unwired: 6 in, 1 out]
            n179 = Bundle By Name(cluster=w358, "SyncEdge"=w363) -> (w357:refnum<class "MultiHarp150.lvclass">)
            n180 = local read "Init Program"() -> (w356:bool)
            n181 = case shown="Faux" w356 {
              tunnel: [w369 w372] -> w361
              tunnel: w360 -> [w368 w371]
              tunnel: [w367 w371] -> w359
              tunnel: w357 -> [w366 w372]
              frame False {
                w370 = T13 1 items=["UpdateClassData", "UpdateMainClass"] ("Menu déroulant")
                n182 = call-dynamic "SetClassQueueMessage.vi"("ErrorIn(No Error)"=w368, "Menu déroulant"=w370, "DefaultDev.lvclass"=w366) -> ("sortie d'erreur"=w367:errorcluster, "DefaultDev.lvclass Out"=w369:refnum<class "MultiHarp150.lvclass">)  [unwired: 7 in]
              }
              frame True {
              }
            }
          }
          event "SyncLevel": Value Change {
            w377 = T13 1 items=["UpdateClassData", "UpdateMainClass"] ("Menu déroulant")
            n183 = event-data() -> ("NewVal"=w378:i32)  [unwired: 1 in]
            n184 = local read "SyncEdge"() -> (w379:i32)
            n185 = local read "DevIdx"() -> (w382:i32)
            n186 = call <userlib>:"MH_SetSyncEdgeTrg.vi"("error in (no error)"=w380, "edge"=w379, "level"=w378, "devidx"=w382) -> ("error out"=w374:errorcluster)  [unwired: 6 in, 1 out]
            n187 = Bundle By Name(cluster=w381, "SyncLevel"=w378) -> (w376:refnum<class "MultiHarp150.lvclass">)
            n188 = call-dynamic "SetClassQueueMessage.vi"("ErrorIn(No Error)"=w374, "Menu déroulant"=w377, "DefaultDev.lvclass"=w376) -> ("sortie d'erreur"=w373:errorcluster, "DefaultDev.lvclass Out"=w375:refnum<class "MultiHarp150.lvclass">)  [unwired: 7 in]
          }
          event "SyncDeadTime": Value Change {
            n189 = event-data() -> ("NewVal"=w386:i32)  [unwired: 1 in]
            n190 = local read "UseDeadTime"() -> (w385:bool)
            n191 = local read "DevIdx"() -> (w394:i32)
            n192 = Boolean To (0,1)(Boolean=w385) -> (0, 1=w387:i16)
            n193 = To Long Integer(number=w387) -> (32bit integer=w384:i32)
            n194 = call <userlib>:"MH_SetSyncDeadTime.vi"("error in (no error)"=w392, "deadtime"=w386, "on"=w384, "devidx"=w394) -> ("error out"=w389:errorcluster)  [unwired: 6 in, 1 out]
            n195 = Bundle By Name(cluster=w393, "SyncDeadTime"=w386) -> (w391:refnum<class "MultiHarp150.lvclass">)
            n196 = local read "Init Program"() -> (w383:bool)
            n197 = case shown="Faux" w383 {
              tunnel: w391 -> [w398 w400]
              tunnel: [w397 w400] -> w390
              tunnel: w389 -> [w396 w401]
              tunnel: [w395 w401] -> w388
              frame False {
                w399 = T13 1 items=["UpdateClassData", "UpdateMainClass"] ("Menu déroulant")
                n198 = call-dynamic "SetClassQueueMessage.vi"("ErrorIn(No Error)"=w396, "Menu déroulant"=w399, "DefaultDev.lvclass"=w398) -> ("sortie d'erreur"=w395:errorcluster, "DefaultDev.lvclass Out"=w397:refnum<class "MultiHarp150.lvclass">)  [unwired: 7 in]
              }
              frame True {
              }
            }
          }
          event "Channels": Value Change {
            w415 = T13 1 items=["UpdateClassData", "UpdateMainClass"] ("Menu déroulant")
            n199 = event-data() -> ("OldVal"=w412:T8[], "NewVal"=w411:T8[])  [unwired: 1 in, 4 out]
            n200 = call <userlib>:"MH_SetInputChannels.vi"("error in (no error)"=w410, "Channels new"=w411, "Channels old"=w412) -> ("error out"=w409:errorcluster, "SetInpChan"=w405:T1[], "Channels"=w406:T8[])  [unwired: 6 in]
            n201 = Bundle By Name(cluster=w408, "Channels"=w406) -> (w407:refnum<class "MultiHarp150.lvclass">)
            n202 = local write "Channels"(w406) -> ()
            n203 = property on="SetInpChan" class="Tabl (strict)"(error in=w409, "Val(Sgnl)"=w405) -> (error out=w404:errorcluster)  [unwired: 1 in, 1 out]
            n204 = call "SetHistDataName.vi"("error in (no error)"=w404, "SetInpChan"=w405, "Channels"=w406, "MultiHarp150.lvclass"=w407) -> ("error out"=w403:errorcluster, "MultiHarp150.lvclass Out"=w402:refnum<class "MultiHarp150.lvclass">)  [unwired: 6 in]
            n205 = call-dynamic "SetClassQueueMessage.vi"("ErrorIn(No Error)"=w403, "Menu déroulant"=w415, "DefaultDev.lvclass"=w402) -> ("sortie d'erreur"=w413:errorcluster, "DefaultDev.lvclass Out"=w414:refnum<class "MultiHarp150.lvclass">)  [unwired: 7 in]
          }
          event "Stats Ch": Value Change {
            n206 = event-data() -> ("NewVal"=w418:u16)  [unwired: 1 in, 5 out]
            n207 = Build Array(w418) -> (w417:u16[])
            n208 = property on="AllHistoStats" class="Tabl (strict)"("Index Values"=w417) -> ()  [unwired: 2 in, 2 out]
          }
          event "SetInpChan": Value Change {
            n209 = event-data() -> ("NewVal"=w426:T1[])  [unwired: 1 in]
            n210 = local read "Channels"() -> (w429:T8[])
            n211 = local read "DevIdx"() -> (w431:i32)
            n212 = Empty Array?(array=w429) -> (empty?=w428:bool)
            n213 = Select(t=T8[] [{"Name"="Ch.1", "Enable"=FALSE, "Edge"=0, "Level"=-150, "Offset"=0, "UseDeadTime"=FALSE, "DeadTime"=800}, {"Name"="Ch.2", "Enable"=FALSE, "Edge"=0, "Level"=-150, "Offset"=0, "UseDeadTime"=FALSE, "DeadTime"=800}, {"Name"="Ch.3", "Enable"=FALSE, "Edge"=0, "Level"=-150, "Offset"=0, "UseDeadTime"=FALSE, "DeadTime"=800}, {"Name"="Ch.4", "Enable"=FALSE, "Edge"=0, "Level"=-150, "Offset"=0, "UseDeadTime"=FALSE, "DeadTime"=800}] ("Channels"), s=w428, f=w429) -> (s? t:f=w422:T8[])
            n214 = case shown="Vrai" w428 {
              tunnel: w427 -> [w441 w444]
              tunnel: [w441 w443] -> w423
              tunnel: w422 -> [_ w442]
              frame False {
              }
              frame True {
                n215 = Bundle By Name(cluster=w444, "Channels"=w442) -> (w443:refnum<class "MultiHarp150.lvclass">)
                n216 = local write "Channels"(w442) -> ()
              }
            }
            n217 = for {
              tunnel: w426 -> [w448] mode=indexing
              shift-right: [w452] -> w432
              shift-left: w424 -> [w451]
              tunnel: w422 -> [w450]
              tunnel: w431 -> [w449]
              n218 = Unbundle By Name(w448) -> ("Cmds"=w447:T2[], "Channel"=w445:i32)
              n219 = Index Array(array=w450, index=w445) -> (element=w446:T8)
              n220 = for {
                tunnel: w445 -> [w458]
                tunnel: w446 -> [w455]
                tunnel: w449 -> [w454]
                tunnel: w447 -> [w453] mode=indexing
                shift-right: [w457] -> w452
                shift-left: w451 -> [w456]
                n221 = case shown="\"SetInpChanDeadTime\"" w453 {
                  tunnel: w458 -> [_ w463 w467 w473 w483]
                  tunnel: [w459 w460 w470 w475 w481] -> w457
                  tunnel: w456 -> [w459 w461 w469 w472 w482]
                  tunnel: w455 -> [_ w465 w471 w480 w487]
                  tunnel: w454 -> [_ w464 w466 w474 w486]
                  frame Default {
                  }
                  frame "SetInpChanEnable" {
                    n222 = Unbundle By Name(w465) -> ("Enable"=w462:bool)
                    n223 = call <userlib>:"MH_SetInputChannelEnable.vi"("error in (no error)"=w461, "enable"=w462, "channel"=w463, "devidx"=w464) -> ("error out"=w460:errorcluster)  [unwired: 6 in, 1 out]
                  }
                  frame "SetInpChanOffset" {
                    n224 = Unbundle By Name(w471) -> ("Offset"=w468:i32)
                    n225 = call <userlib>:"MH_SetInputChannelOffset.vi"("error in (no error)"=w469, "Offset"=w468, "channel"=w467, "devidx"=w466) -> ("error out"=w470:errorcluster)  [unwired: 6 in, 1 out]
                  }
                  frame "SetInpChanDeadTime" {
                    n226 = Unbundle By Name(w480) -> ("UseDeadTime"=w479:bool, "DeadTime"=w476:i32)
                    n227 = Boolean To (0,1)(Boolean=w479) -> (0, 1=w478:i16)
                    n228 = To Long Integer(number=w478) -> (32bit integer=w477:i32)
                    n229 = call <userlib>:"MH_SetInputDeadTime.vi"("channel"=w473, "error in (no error)"=w472, "deadtime"=w476, "on"=w477, "devidx"=w474) -> ("error out"=w475:errorcluster)  [unwired: 5 in, 1 out]
                  }
                  frame "SetInpChanTrg" {
                    n230 = Unbundle By Name(w487) -> ("Level"=w485:i32, "Edge"=w484:i32)
                    n231 = call <userlib>:"MH_SetInputEdgeTrg.vi"("channel"=w483, "error in (no error)"=w482, "edge"=w484, "level"=w485, "devidx"=w486) -> ("error out"=w481:errorcluster)  [unwired: 5 in, 1 out]
                  }
                }
              }
            }
            n232 = local read "Init Program"() -> (w419:bool)
            n233 = case shown="Vrai" w419 {
              tunnel: w424 -> [w433 w440]
              tunnel: w423 -> [w434 w439]
              tunnel: w422 -> [_ w438]
              tunnel: [w434 w437] -> w421
              tunnel: [w433 w436] -> w420
              frame False {
              }
              frame True {
                n234 = call "SetHistDataName.vi"("ForceSet"=TRUE, "error in (no error)"=w440, "Channels"=w438, "MultiHarp150.lvclass"=w439) -> ("error out"=w436:errorcluster, "MultiHarp150.lvclass Out"=w437:refnum<class "MultiHarp150.lvclass">)  [unwired: 6 in]
              }
            }
            n235 = Merge Errors(w420, w432) -> (w425:errorcluster)
          }
          event "Acqu. Time (ms)": Value Change {
            w492 = T13 1 items=["UpdateClassData", "UpdateMainClass"] ("Menu déroulant")
            n236 = event-data() -> ("NewVal"=w493:i32)  [unwired: 1 in, 5 out]
            n237 = Bundle By Name(cluster=w494, "AcquTime(ms)"=w493) -> (w491:refnum<class "MultiHarp150.lvclass">)
            n238 = call-dynamic "SetClassQueueMessage.vi"("ErrorIn(No Error)"=w488, "Menu déroulant"=w492, "DefaultDev.lvclass"=w491) -> ("sortie d'erreur"=w489:errorcluster, "DefaultDev.lvclass Out"=w490:refnum<class "MultiHarp150.lvclass">)  [unwired: 7 in]
          }
          event "Binning": Value Change {
            n239 = event-data() -> ("NewVal"=w504:T4)  [unwired: 1 in]
            n240 = To Long Integer(number=w504) -> (32bit integer=w500:i32)
            n241 = local read "DevIdx"() -> (w498:i32)
            n242 = Unbundle By Name(w496) -> ("Mode"=w495:T7)
            n243 = case shown="1, Par défaut" w495 {
              tunnel: w496 -> [w506 w519]
              tunnel: w505 -> [w507 w518]
              tunnel: [w506 w517] -> w503
              tunnel: w500 -> [_ w515]
              tunnel: [w507 w513] -> w499
              tunnel: w498 -> [_ w512]
              frame 1, Default {
                # "Prop Not ValiD in g(t) MODE"
              }
              frame 0 {
                n244 = call <userlib>:"MH_SetBinning.vi"("error in (no error)"=w518, "Binning"=w515, "devidx"=w512) -> ("error out"=w516:errorcluster, "return type"=w514:i32)  [unwired: 7 in]
                n245 = call <userlib>:"MH_GetBaseResolution.vi"("error in (no error)"=w516, "devidx"=w512) -> ("error out"=w513:errorcluster, "binsteps"=→"binsteps":i32, "resolution"=w510:dbl)  [unwired: 6 in, 1 out]
                n246 = Divide(x=w510, y=1000.0) -> (x/y=w509:dbl)
                n247 = Bundle By Name(cluster=w519, "Binning"=w514, "Resolution (ns)"=w509) -> (w517:refnum<class "MultiHarp150.lvclass">)
              }
            }
            n248 = local read "Init Program"() -> (w497:bool)
            n249 = case shown="Faux" w497 {
              tunnel: w503 -> [w523 w526]
              tunnel: [w522 w526] -> w502
              tunnel: [w521 w525] -> w501
              tunnel: w499 -> [w520 w525]
              frame False {
                w524 = T13 1 items=["UpdateClassData", "UpdateMainClass"] ("Menu déroulant")
                n250 = call-dynamic "SetClassQueueMessage.vi"("ErrorIn(No Error)"=w520, "Menu déroulant"=w524, "DefaultDev.lvclass"=w523) -> ("sortie d'erreur"=w521:errorcluster, "DefaultDev.lvclass Out"=w522:refnum<class "MultiHarp150.lvclass">)  [unwired: 7 in]
              }
              frame True {
              }
            }
          }
          event "HistoLength": Value Change {
            n251 = event-data() -> ("NewVal"=w534:T5)  [unwired: 1 in]
            n252 = local read "DevIdx"() -> (w536:i32)
            n253 = Unbundle By Name(w528) -> ("Mode"=w527:T7)
            n254 = case shown="0" w527 {
              tunnel: w536 -> [_ w549]
              tunnel: w528 -> [w538 w548]
              tunnel: w535 -> [w537 w547]
              tunnel: w534 -> [_ w546]
              tunnel: [w538 w545] -> w533
              tunnel: [w537 w539] -> w529
              frame 1, Default {
                # "Prop Not ValiD in g(t) MODE"
              }
              frame 0 {
                n255 = To Long Integer(number=w546) -> (32bit integer=w544:i32)
                n256 = call <userlib>:"MH_SetHistoLen.vi"("error in (no error)"=w547, "lencode"=w544, "devidx"=w549) -> ("error out"=w540:errorcluster, "actuallen"=w542:i32)  [unwired: 6 in, 1 out]
                n257 = for {
                  N: w542 -> [_]
                  tunnel: [w550] -> w541 mode=indexing
                  i -> [w551]
                  n258 = To Double Precision Float(number=w551) -> (double precision float=w550:dbl)
                }
                n259 = property class="MultiHarp150.lvclass"(reference=w548, error in=w540, "Accessor:ScanTable"=w541) -> (reference out=w543:refnum<class "MultiHarp150.lvclass">, error out=w539:errorcluster)
                n260 = Bundle By Name(cluster=w543, "HistoLength"=w546, "Actual_H_Lenght(bin)"=w542) -> (w545:refnum<class "MultiHarp150.lvclass">)
              }
            }
            n261 = local read "Init Program"() -> (w530:bool)
            n262 = case shown="Faux" w530 {
              tunnel: w533 -> [w555 w558]
              tunnel: [w554 w558] -> w532
              tunnel: w529 -> [w553 w557]
              tunnel: [w552 w557] -> w531
              frame False {
                w556 = T13 1 items=["UpdateClassData", "UpdateMainClass"] ("Menu déroulant")
                n263 = call-dynamic "SetClassQueueMessage.vi"("ErrorIn(No Error)"=w553, "Menu déroulant"=w556, "DefaultDev.lvclass"=w555) -> ("sortie d'erreur"=w552:errorcluster, "DefaultDev.lvclass Out"=w554:refnum<class "MultiHarp150.lvclass">)  [unwired: 7 in]
              }
              frame True {
              }
            }
          }
          event "AcqOffset (ns)": Value Change {
            n264 = event-data() -> ("NewVal"=w561:i32)  [unwired: 1 in]
            n265 = Unbundle By Name(w560) -> ("Mode"=w559:T7)
            n266 = case shown="1, Par défaut" w559 {
              tunnel: w560 -> [w569 w574]
              tunnel: w567 -> [w568 w573]
              tunnel: [w569 w572] -> w566
              tunnel: [w568 w571] -> w564
              tunnel: w561 -> [_ w570]
              frame 1, Default {
                # "Prop Not ValiD in g(t) MODE"
              }
              frame 0 {
                n267 = local read "DevIdx"() -> (w575:i32)
                n268 = Bundle By Name(cluster=w574, "HistoOffset(ns)"=w570) -> (w572:refnum<class "MultiHarp150.lvclass">)
                n269 = call <userlib>:"MH_SetOffset.vi"("error in (no error)"=w573, "Offset"=w570, "devidx"=w575) -> ("error out"=w571:errorcluster)  [unwired: 7 in, 1 out]
              }
            }
            n270 = local read "Init Program"() -> (w562:bool)
            n271 = case shown="Faux" w562 {
              tunnel: w566 -> [w579 w582]
              tunnel: [w578 w582] -> w565
              tunnel: w564 -> [w577 w581]
              tunnel: [w576 w581] -> w563
              frame False {
                w580 = T13 1 items=["UpdateClassData", "UpdateMainClass"] ("Menu déroulant")
                n272 = call-dynamic "SetClassQueueMessage.vi"("ErrorIn(No Error)"=w577, "Menu déroulant"=w580, "DefaultDev.lvclass"=w579) -> ("sortie d'erreur"=w576:errorcluster, "DefaultDev.lvclass Out"=w578:refnum<class "MultiHarp150.lvclass">)  [unwired: 7 in]
              }
              frame True {
              }
            }
          }
          event "Stop Ovl.": Value Change {
            w590 = T13 1 items=["UpdateClassData", "UpdateMainClass"] ("Menu déroulant")
            n273 = event-data() -> ("NewVal"=w585:bool)  [unwired: 1 in]
            n274 = local read "DevIdx"() -> (w592:i32)
            n275 = Unbundle By Name(w584) -> ("Mode"=w583:T7)
            n276 = case shown="1, Par défaut" w583 {
              tunnel: w592 -> [w597 _]
              tunnel: w591 -> [w596 w598]
              tunnel: [w595 w598] -> w587
              tunnel: w585 -> [w594 _]
              frame 0 {
                n277 = local read "OvlLevel"() -> (w593:u32)
                n278 = call <userlib>:"MH_SetStopOverflow.vi"("error in (no error)"=w596, "stopcount"=w593, "StopOnOverflow"=w594, "devidx"=w597) -> ("error out"=w595:errorcluster)  [unwired: 6 in, 1 out]
              }
              frame 1, Default {
                # "Prop Not ValiD in g(t) MODE"
              }
            }
            n279 = Bundle By Name(cluster=w584, "Stop Ovl."=w585) -> (w589:refnum<class "MultiHarp150.lvclass">)
            n280 = call-dynamic "SetClassQueueMessage.vi"("ErrorIn(No Error)"=w587, "Menu déroulant"=w590, "DefaultDev.lvclass"=w589) -> ("sortie d'erreur"=w586:errorcluster, "DefaultDev.lvclass Out"=w588:refnum<class "MultiHarp150.lvclass">)  [unwired: 7 in]
          }
          event "OvlLevel": Value Change {
            w608 = T13 1 items=["UpdateClassData", "UpdateMainClass"] ("Menu déroulant")
            n281 = event-data() -> ("NewVal"=w604:u32)  [unwired: 1 in]
            n282 = Unbundle By Name(w600) -> ("Mode"=w599:T7)
            n283 = case shown="0" w599 {
              tunnel: w609 -> [w610 w614]
              tunnel: [w610 w613] -> w605
              tunnel: w604 -> [_ w612]
              frame 1, Default {
              }
              frame 0 {
                n284 = local read "UseDeadTime"() -> (w611:bool)
                n285 = local read "DevIdx"() -> (w615:i32)
                n286 = call <userlib>:"MH_SetStopOverflow.vi"("error in (no error)"=w614, "stopcount"=w612, "StopOnOverflow"=w611, "devidx"=w615) -> ("error out"=w613:errorcluster)  [unwired: 6 in, 1 out]
              }
            }
            n287 = Bundle By Name(cluster=w600, "OvlLevel"=w604) -> (w607:refnum<class "MultiHarp150.lvclass">)
            n288 = local read "Init Program"() -> (w603:bool)
            n289 = call-dynamic "SetClassQueueMessage.vi"("ErrorIn(No Error)"=w605, "Menu déroulant"=w608, "DefaultDev.lvclass"=w607) -> ("sortie d'erreur"=w602:errorcluster, "DefaultDev.lvclass Out"=w606:refnum<class "MultiHarp150.lvclass">)  [unwired: 7 in]
            n290 = case shown="Vrai" w603 {
              tunnel: w602 -> [w616 w619]
              tunnel: [w616 w617] -> w601
              frame False {
              }
              frame True {
                n291 = property on="MH Tabs" class="Onglet (strict)"(error in=w619, "Value"=enum32{"Main", "Settings", "Channels"}."Main" ("MH Tabs")) -> (error out=w617:errorcluster)  [unwired: 1 in, 1 out]
                n292 = local write "Init Program"(FALSE ("Init Program")) -> ()
                n293 = local write "Con/Disc."(TRUE ("Init Program")) -> ()
              }
            }
          }
          event "AquireHist": Value Change {
            n294 = event-data() -> ("NewVal"=w626:bool)  [unwired: 1 in]
            n295 = case shown="Vrai" w626 {
              tunnel: w627 -> [w630 w658]
              tunnel: w623 -> [_ w634]
              tunnel: w622 -> [_ w644]
              tunnel: [w630 w631] -> w628
              tunnel: w625 -> [w629 w652]
              tunnel: [w629 w651] -> w624
              frame False {
              }
              frame True {
                w632 = FALSE ("Rate Graph")
                n296 = property class="MultiHarp150.lvclass"(reference=w658, error in=w652) -> (reference out=w631:refnum<class "MultiHarp150.lvclass">, error out=w642:errorcluster, "Accessor:Function"=w650:string, "Accessor:InstrumentName"=w648:string)
                n297 = local write "Read Cont."(w632) -> ()
                n298 = local write "Rate Graph"(w632) -> ()
                n299 = local write "RtGrphAct"(w632) -> ()
                n300 = local read "Graph #"() -> (w635:i32)
                n301 = local read "Save Data"() -> (w641:bool)
                n302 = local read "Clear Graph"() -> (w636:bool)
                n303 = Concatenate Strings(w650, "@" ("chaîne"), w648) -> (w637:string)
                n304 = Bundle By Name(cluster=cluster{"Message":string, "Data":variant, i32} {"Message"="ClearGraph", "Data"=variant, 0} ("élément"), "Data"=w635) -> (w638:cluster{"Message":string, "Data":variant, i32})
                n305 = Unbundle By Name(w631) -> ()  [unwired: 1 out]
                n306 = case shown="Vrai" w636 {
                  tunnel: [w661 w664] -> w645
                  tunnel: w644 -> [w660 w669]
                  tunnel: [w660 w662] -> w643
                  tunnel: w642 -> [w661 w668]
                  tunnel: w638 -> [_ w667]
                  tunnel: w634 -> [w659 w666]
                  tunnel: [w659 w663] -> w633
                  frame False {
                  }
                  frame True {
                    n307 = Enqueue Element(queue=w669, element=w667, error in (no error)=w668) -> (queue out=w662:refnum<queue>, error out=w665:errorcluster)  [unwired: 1 in, 1 out]
                    n308 = Generate User Event(user event=w666, event data cluster=w662, error in=w665) -> (user event out=w663:refnum<user-event>, error out=w664:errorcluster)  [unwired: 1 in]
                  }
                }
                n309 = Bundle(w637, "Save Data"=w641) -> (w640:cluster{string, "Save Data":bool})  [unwired: 1 in]
                n310 = To Variant(anything=w640) -> (Variant=w655:variant)
                n311 = Wait (ms)(milliseconds to wait=u32 200 ("attente (ms)")) -> (millisecond timer value=w647:u32)
                n312 = flat-sequence {
                  tunnel: w647 -> [_]
                  frame #0 {
                    n313 = local write "AquireHist"(FALSE) -> ()
                  }
                }
                n314 = Bundle By Name(cluster=cluster{"Message":string, "Data":variant, i32} {"Message"="ArrayDevAcqSetup", "Data"=variant, 0} ("élément"), "Data"=w655) -> (w654:cluster{"Message":string, "Data":variant, i32})
                n315 = Enqueue Element(queue=w643, element=w654, error in (no error)=w645) -> (queue out=w657:refnum<queue>, error out=w653:errorcluster)  [unwired: 1 in, 1 out]
                n316 = Generate User Event(user event=w633, event data cluster=w657, error in=w653) -> (error out=w651:errorcluster)  [unwired: 1 in, 1 out]
              }
            }
          }
          event "Stop": Value Change {
            n317 = event-data() -> ("NewVal"=w671:bool)  [unwired: 1 in, 5 out]
            n318 = case shown="Faux" w671 {
              tunnel: w675 -> [w677 w700]
              tunnel: w674 -> [w678 w699]
              tunnel: [w678 w698] -> w673
              tunnel: [w677 w680] -> w672
              frame False {
              }
              frame True {
                n319 = local read "Panel Refresh"() -> (w697:u32)
                n320 = local read "HistoLength"() -> (w684:T5)
                n321 = local read "Stop Ovl."() -> (w696:bool)
                n322 = local read "OvlLevel"() -> (w695:u32)
                n323 = local read "Binning"() -> (w694:T4)
                n324 = local read "SyncLevel"() -> (w693:i32)
                n325 = local read "SyncEdge"() -> (w692:i32)
                n326 = local read "SyncDivider"() -> (w691:i32)
                n327 = local read "SyncDeadTime"() -> (w690:i32)
                n328 = local read "UseDeadTime"() -> (w689:bool)
                n329 = local read "SyncOffset"() -> (w688:i32)
                n330 = local read "Acqu. Time (ms)"() -> (w682:i32)
                n331 = local read "Channels"() -> (w687:T8[])
                n332 = local read "Mode"() -> (w686:T7)
                n333 = local read "Ref Source"() -> (w685:T6)
                n334 = local read "AcqOffset (ns)"() -> (w683:i32)
                n335 = Bundle By Name(cluster=w699, "Panel Refresh"=w697, "HistoLength"=w684, "Stop Ovl."=w696, "OvlLevel"=w695, "Binning"=w694, "SyncLevel"=w693, "SyncEdge"=w692, "SyncDivider"=w691, "SyncDeadTime"=w690, "UseDeadTime"=w689, "SyncOffset"=w688, "Channels"=w687, "Mode"=w686, "refsource"=w685, "HistoOffset(ns)"=w683, "AcquTime(ms)"=w682) -> (w698:refnum<class "MultiHarp150.lvclass">)
                n336 = call "SaveChildClassValues.vi"("error in (no error)"=w700, "MultiHarp150 en entrée"=w698) -> ("error out"=w679:errorcluster)  [unwired: 8 in, 1 out]
                n337 = local read "DevIdx"() -> (w681:i32)
                n338 = call <userlib>:"MH_CloseDevice.vi"("error in (no error)"=w679, "devidx"=w681) -> ("error out"=w680:errorcluster)  [unwired: 8 in, 1 out]
              }
            }
          }
          event "Con/Disc.": Value Change {
            n339 = event-data() -> ("NewVal"=w701:bool)  [unwired: 1 in, 5 out]
            n340 = case shown="Vrai" w701 {
              tunnel: [w708 w711] -> w704
              tunnel: w702 -> [w707 w712]
              frame False {
                n341 = local read "DevIdx"() -> (w709:i32)
                n342 = call <userlib>:"MH_CloseDevice.vi"("error in (no error)"=w707, "devidx"=w709) -> ("error out"=w708:errorcluster)  [unwired: 8 in, 1 out]
                n343 = local write "Read Cont."(FALSE ("Read Cont.")) -> ()
              }
              frame True {
                n344 = property on="Init Program" class="Bool (strict)"(error in=w712, "Val(Sgnl)"=TRUE ("Valeur (Signalisation)")) -> (error out=w711:errorcluster)  [unwired: 1 in, 1 out]
              }
            }
          }
          event "Rd.Cnt\nAcqu.": Value Change {
            w721 = T13 1 items=["UpdateClassData", "UpdateMainClass", "UpdateDataBind", "ReInitDevice"] ("Menu déroulant")
            n345 = event-data() -> ("NewVal"=w727:bool)  [unwired: 1 in, 5 out]
            n346 = case shown="Faux" w727 {
              tunnel: w726 -> [w729 w740]
              tunnel: w725 -> [w731 w741]
              tunnel: [w731 w741] -> w714
              tunnel: [w732 w742] -> w722
              tunnel: [T11."DisAndGrayed" ("Énum") T11."Enable" ("Énum")] -> w716
              frame True {
                n347 = Bundle By Name(cluster=w729, "Functions"=MultiHarp150_Func."ReadCount (Ph)") -> (w732:refnum<class "MultiHarp150.lvclass">)
              }
              frame False {
                w738 = T7 2 items=["HIST"=0, "T2"=2, "T3"=3] ("y")
                n348 = Unbundle By Name(w740) -> ("Mode"=w739:T7)
                n349 = Equal?(x=w739, y=w738) -> (x = y?=w736:bool)
                n350 = Select(t=MultiHarp150_Func."ReadT2 (Ph)" ("Functions"), s=w736, f=MultiHarp150_Func."ReadHistogram (Ph)" ("Functions")) -> (s? t:f=w733:T10)
                n351 = Bundle By Name(cluster=w740, "Functions"=w733) -> (w742:refnum<class "MultiHarp150.lvclass">)
              }
            }
            n352 = control-ref of="AquireHist"() -> (w713:refnum<vi>)
            n353 = local read "Channels"() -> (w718:T8[])
            n354 = call <userlib>:"SetCtrlPropGenSgl.vi"("Error in"=w714, "Énum"=w716, "Controls"=w713) -> ("Error out"=w715:errorcluster)  [unwired: 3 in, 1 out]
            n355 = call "SetHistDataName.vi"("ForceSet"=TRUE, "error in (no error)"=w715, "Channels"=w718, "MultiHarp150.lvclass"=w722) -> ("error out"=w723:errorcluster, "MultiHarp150.lvclass Out"=w724:refnum<class "MultiHarp150.lvclass">)  [unwired: 6 in]
            n356 = call-dynamic "SetClassQueueMessage.vi"("ErrorIn(No Error)"=w723, "Menu déroulant"=w721, "DefaultDev.lvclass"=w724) -> ("sortie d'erreur"=w720:errorcluster, "DefaultDev.lvclass Out"=w719:refnum<class "MultiHarp150.lvclass">)  [unwired: 7 in]
          }
        }
      }
    }
    frame Error {
    }
  }
  "error out" <- w5
  "MultiHarp150.lvclass Out" <- w3
